vi "06-TemperaturaMedia.vi"() -> ()   [LabVIEW 2014]
panel:
  in  "Temp Scale":bool
  out "Temp historico":cluster{dbl, "Thermometer":dbl}(graph)
  in  "Power":bool
  # "ON"
  # "OFF"
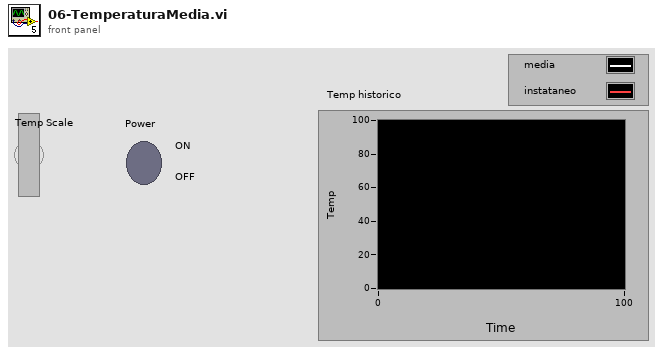
[diagram p1: front panel]
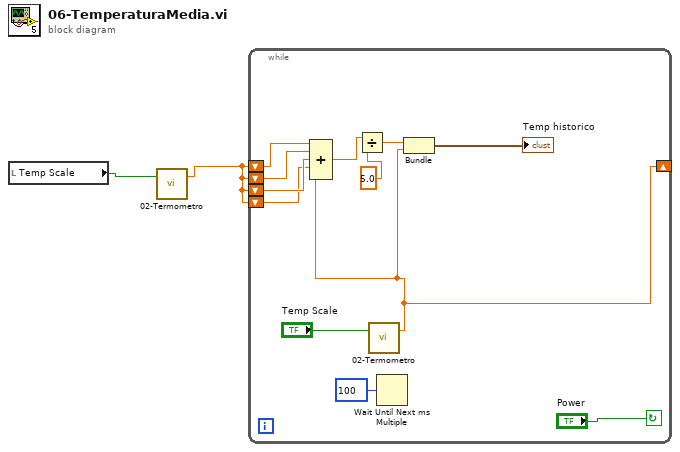
[diagram p0: block diagram]
diagram:
  n1 = local read "Temp Scale"() -> (w1:bool)
  n2 = call "02-Termometro.vi"("Temp Scale"=w1) -> ("Thermometer"=w2:dbl)  [unwired: 2 in]
  n3 = while {
    shift-right: [w3] -> _
    shift-left: w2 -> [w11]
    shift-left: w2 -> [w10]
    shift-left: w2 -> [w9]
    shift-left: w2 -> [w8]
    stop <- "Power" continue-if-true
    n4 = call "02-Termometro.vi"("Temp Scale"="Temp Scale") -> ("Thermometer"=w3:dbl)  [unwired: 2 in]
    n5 = Compound Arithmetic op=ADD(w11, w10, w9, w8, w3) -> (w7:dbl)
    n6 = Divide(x=w7, y=5.0) -> (x/y=w5:dbl)
    n7 = Wait Until Next ms Multiple(millisecond multiple=u32 100) -> ()  [unwired: 1 out]
    n8 = Bundle(w5, "Thermometer"=w3) -> (→"Temp historico":cluster{dbl, "Thermometer":dbl})  [unwired: 1 in]
  }
